vi "mislanius_time_add.vi"(8 "error in (no error)":errorcluster, 10 "Cluster out":T1={"connection reference"=refnum, "Net Avai time (Min)"=0, "pLAN dATE datA"=[], "Data by plan date, shift, product"=[], "BreakDownd Data"=[], "Raw rejection Data"=[], "mislanius times shift 1"={"Lunch Time From"=timestamp(0 s since 1904-01-01), "Lunch Time To"=timestamp(0 s since 1904-01-01), "Tea Time From"=timestamp(0 s since 1904-01-01), "Tea Time To"=timestamp(0 s since 1904-01-01), "Clean Time From"=timestamp(0 s since 1904-01-01), "Clean Time To"=timestamp(0 s since 1904-01-01), "Meeting Time From"=timestamp(0 s since 1904-01-01), "Meeting Time To"=timestamp(0 s since 1904-01-01), "Dev/Other Time From"=timestamp(0 s since 1904-01-01), "Dev/Other Time To"=timestamp(0 s since 1904-01-01), "Meeting"=FALSE, "Dev/Other"=TRUE}, "mislanius times shift 2"={"Lunch Time From"=timestamp(0 s since 1904-01-01), "Lunch Time To"=timestamp(0 s since 1904-01-01), "Tea Time From"=timestamp(0 s since 1904-01-01), "Tea Time To"=timestamp(0 s since 1904-01-01), "Clean Time From"=timestamp(0 s since 1904-01-01), "Clean Time To"=timestamp(0 s since 1904-01-01), "Meeting Time From"=timestamp(0 s since 1904-01-01), "Meeting Time To"=timestamp(0 s since 1904-01-01), "Dev/Other Time From"=timestamp(0 s since 1904-01-01), "Dev/Other Time To"=timestamp(0 s since 1904-01-01), "Meeting"=FALSE, "Dev/Other"=TRUE}} {"mislanius times shift 2"."Lunch Time From" format="%<%.X %x>T"; "mislanius times shift 2"."Lunch Time To" format="%<%.X %x>T"; "mislanius times shift 2"."Tea Time From" format="%<%.X %x>T"; "mislanius times shift 2"."Tea Time To" format="%<%.X %x>T"; "mislanius times shift 2"."Clean Time From" format="%<%.X %x>T"; "mislanius times shift 2"."Clean Time To" format="%<%.X %x>T"; "mislanius times shift 2"."Meeting Time From" format="%<%.X %x>T"; "mislanius times shift 2"."Meeting Time To" format="%<%.X %x>T"; "mislanius times shift 2"."Dev/Other Time From" format="%<%.X %x>T"; "mislanius times shift 2"."Dev/Other Time To" format="%<%.X %x>T"; "mislanius times shift 1"."Lunch Time From" format="%<%.X %x>T"; "mislanius times shift 1"."Lunch Time To" format="%<%.X %x>T"; "mislanius times shift 1"."Tea Time From" format="%<%.X %x>T"; "mislanius times shift 1"."Tea Time To" format="%<%.X %x>T"; "mislanius times shift 1"."Clean Time From" format="%<%.X %x>T"; "mislanius times shift 1"."Clean Time To" format="%<%.X %x>T"; "mislanius times shift 1"."Meeting Time From" format="%<%.X %x>T"; "mislanius times shift 1"."Meeting Time To" format="%<%.X %x>T"; "mislanius times shift 1"."Dev/Other Time From" format="%<%.X %x>T"; "mislanius times shift 1"."Dev/Other Time To" format="%<%.X %x>T"}, 11 "Shift":string(combo)="2") -> (0 "error out":errorcluster, 2 "Split DT time":u32[](array[numeric]), 3 "Total mis time":i32)   [LabVIEW 2017]
uses:
  Controls/OE_screen_cluster.ctl
  <vilib>/addons/database/Connection.llb/Conn ObjectReference.ctl
  <vilib>/addons/database/NI_Database_API.lvlib
panel:
  out "Lunch time 2":i32
  out "tea time 2":i32
  out "clean time 2":i32
  out "meeting time 2":i32
  out "Dev/other time 2":i32
  out "Dev/other time":i32
  out "meeting time":i32
  out "clean time":i32
  out "tea time":i32
  out "Lunch time":i32
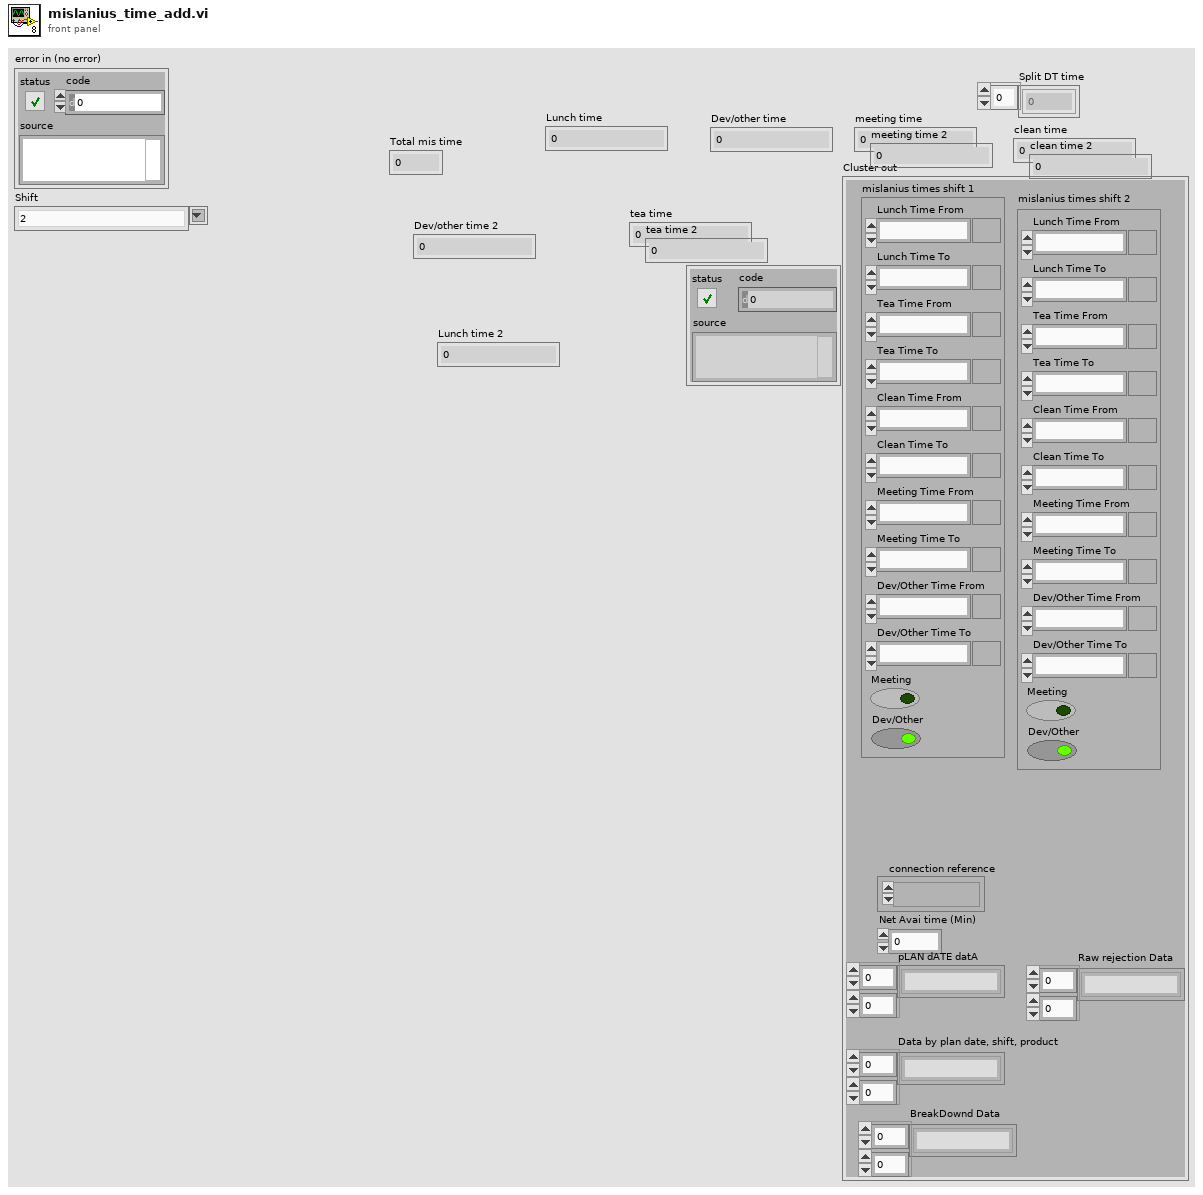
[diagram p1: front panel]
types:
  T1 = typedef "OE_screen_cluster.ctl" = cluster{"connection reference":T2, "Net Avai time (Min)":i32, "pLAN dATE datA":string[][], "Data by plan date, shift, product":string[][], "BreakDownd Data":string[][], "Raw rejection Data":string[][], "mislanius times shift 1":cluster{"Lunch Time From":timestamp, "Lunch Time To":timestamp, "Tea Time From":timestamp, "Tea Time To":timestamp, "Clean Time From":timestamp, "Clean Time To":timestamp, "Meeting Time From":timestamp, "Meeting Time To":timestamp, "Dev/Other Time From":timestamp, "Dev/Other Time To":timestamp, "Meeting":bool, "Dev/Other":bool}, "mislanius times shift 2":cluster{"Lunch Time From":timestamp, "Lunch Time To":timestamp, "Tea Time From":timestamp, "Tea Time To":timestamp, "Clean Time From":timestamp, "Clean Time To":timestamp, "Meeting Time From":timestamp, "Meeting Time To":timestamp, "Dev/Other Time From":timestamp, "Dev/Other Time To":timestamp, "Meeting":bool, "Dev/Other":bool}}
  T2 = typedef "NI_Database_API.lvlib/Conn ObjectReference.ctl" = refnum<k1>
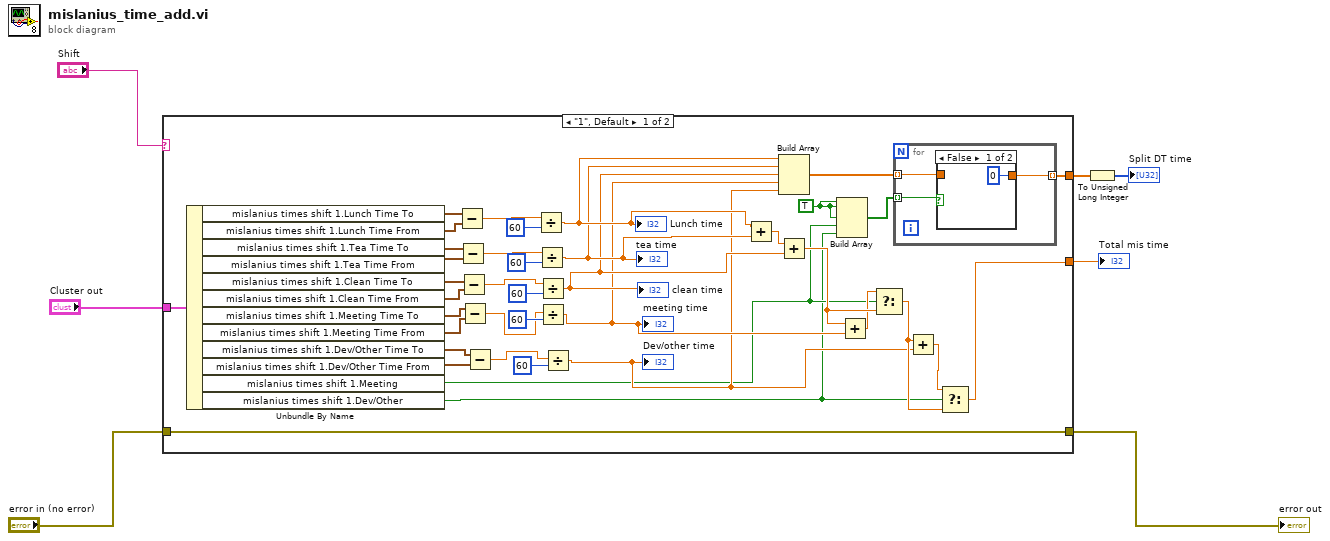
[diagram p0: block diagram]
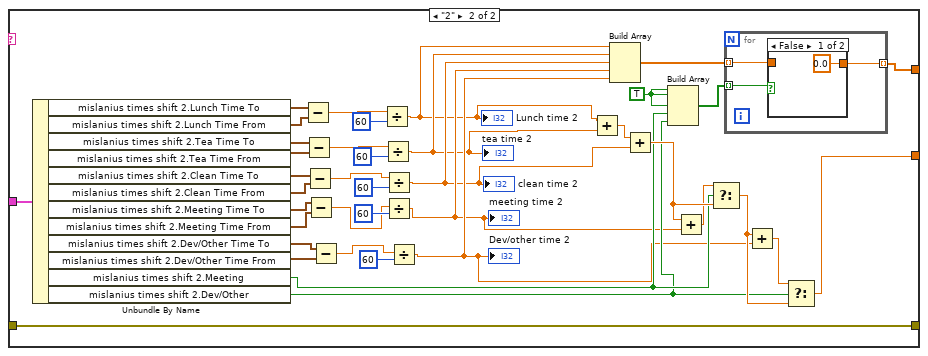
[diagram p3: hidden frame]
diagram:
  n1 = case shown="\"1\", Default" "Shift" {
    tunnel: [w20 w64] -> w7
    tunnel: "Cluster out" -> [w24 w68]
    tunnel: [w19 w63] -> w4
    tunnel: "error in (no error)" -> [w19 w63]
    tunnel: [w8 w60] -> w2
    frame "1", Default {
      w12 = TRUE
      n2 = Unbundle By Name(w24) -> ("mislanius times shift 1.Lunch Time To"=w44:timestamp, "mislanius times shift 1.Lunch Time From"=w43:timestamp, "mislanius times shift 1.Tea Time To"=w42:timestamp, "mislanius times shift 1.Tea Time From"=w41:timestamp, "mislanius times shift 1.Clean Time To"=w37:timestamp, "mislanius times shift 1.Clean Time From"=w36:timestamp, "mislanius times shift 1.Meeting Time To"=w33:timestamp, "mislanius times shift 1.Meeting Time From"=w32:timestamp, "mislanius times shift 1.Dev/Other Time To"=w28:timestamp, "mislanius times shift 1.Dev/Other Time From"=w27:timestamp, "mislanius times shift 1.Meeting"=w11:bool, "mislanius times shift 1.Dev/Other"=w10:bool)
      n3 = Subtract(x=w44, y=w43) -> (x-y=w46:dbl)
      n4 = Subtract(x=w42, y=w41) -> (x-y=w39:dbl)
      n5 = Subtract(x=w37, y=w36) -> (x-y=w34:dbl)
      n6 = Subtract(x=w33, y=w32) -> (x-y=w31:dbl)
      n7 = Subtract(x=w28, y=w27) -> (x-y=w30:dbl)
      n8 = Divide(x=w46, y=60) -> (x/y=w18:dbl)
      "Lunch time" <- w18
      n9 = Divide(x=w39, y=60) -> (x/y=w17:dbl)
      "tea time" <- w17
      n10 = Divide(x=w34, y=60) -> (x/y=w16:dbl)
      "clean time" <- w16
      n11 = Divide(x=w31, y=60) -> (x/y=w15:dbl)
      "meeting time" <- w15
      n12 = Divide(x=w30, y=60) -> (x/y=w14:dbl)
      "Dev/other time" <- w14
      n13 = Add(x=w18, y=w17) -> (x+y=w26:dbl)
      n14 = Build Array(w18, w17, w16, w15, w14) -> (w13:dbl[])
      n15 = Add(x=w26, y=w16) -> (x+y=w25:dbl)
      n16 = Build Array(w12, w12, w12, w11, w10) -> (w9:bool[])
      n17 = Add(x=w25, y=w15) -> (x+y=w23:dbl)
      n18 = Select(t=w23, s=w11, f=w25) -> (s? t:f=w21:dbl)
      n19 = for {
        tunnel: w13 -> [w47] mode=indexing
        tunnel: w9 -> [w49] mode=indexing
        tunnel: [w48] -> w8 mode=indexing
        n20 = case shown="False" w49 {
          tunnel: [0 w51] -> w48
          tunnel: w47 -> [_ w51]
          frame False {
          }
          frame True {
          }
        }
      }
      n21 = Add(x=w21, y=w14) -> (x+y=w22:dbl)
      n22 = Select(t=w22, s=w10, f=w21) -> (s? t:f=w20:dbl)
    }
    frame "2" {
      w61 = TRUE
      n23 = Unbundle By Name(w68) -> ("mislanius times shift 2.Lunch Time To"=w88:timestamp, "mislanius times shift 2.Lunch Time From"=w87:timestamp, "mislanius times shift 2.Tea Time To"=w86:timestamp, "mislanius times shift 2.Tea Time From"=w85:timestamp, "mislanius times shift 2.Clean Time To"=w81:timestamp, "mislanius times shift 2.Clean Time From"=w80:timestamp, "mislanius times shift 2.Meeting Time To"=w77:timestamp, "mislanius times shift 2.Meeting Time From"=w76:timestamp, "mislanius times shift 2.Dev/Other Time To"=w72:timestamp, "mislanius times shift 2.Dev/Other Time From"=w71:timestamp, "mislanius times shift 2.Meeting"=w59:bool, "mislanius times shift 2.Dev/Other"=w58:bool)
      n24 = Subtract(x=w88, y=w87) -> (x-y=w90:dbl)
      n25 = Subtract(x=w86, y=w85) -> (x-y=w83:dbl)
      n26 = Subtract(x=w81, y=w80) -> (x-y=w78:dbl)
      n27 = Subtract(x=w77, y=w76) -> (x-y=w75:dbl)
      n28 = Subtract(x=w72, y=w71) -> (x-y=w74:dbl)
      n29 = Divide(x=w90, y=60) -> (x/y=w53:dbl)
      "Lunch time 2" <- w53
      n30 = Divide(x=w83, y=60) -> (x/y=w54:dbl)
      "tea time 2" <- w54
      n31 = Divide(x=w78, y=60) -> (x/y=w55:dbl)
      "clean time 2" <- w55
      n32 = Divide(x=w75, y=60) -> (x/y=w56:dbl)
      "meeting time 2" <- w56
      n33 = Divide(x=w74, y=60) -> (x/y=w57:dbl)
      "Dev/other time 2" <- w57
      n34 = Add(x=w53, y=w54) -> (x+y=w70:dbl)
      n35 = Build Array(w53, w54, w55, w56, w57) -> (w52:dbl[])
      n36 = Add(x=w70, y=w55) -> (x+y=w69:dbl)
      n37 = Build Array(w61, w61, w61, w59, w58) -> (w62:bool[])
      n38 = Add(x=w69, y=w56) -> (x+y=w67:dbl)
      n39 = Select(t=w67, s=w59, f=w69) -> (s? t:f=w65:dbl)
      n40 = for {
        tunnel: w52 -> [w91] mode=indexing
        tunnel: w62 -> [w93] mode=indexing
        tunnel: [w92] -> w60 mode=indexing
        n41 = case shown="False" w93 {
          tunnel: [0.0 w95] -> w92
          tunnel: w91 -> [_ w95]
          frame False {
          }
          frame True {
          }
        }
      }
      n42 = Add(x=w65, y=w57) -> (x+y=w66:dbl)
      n43 = Select(t=w66, s=w58, f=w65) -> (s? t:f=w64:dbl)
    }
  }
  "Total mis time" <- w7
  "error out" <- w4
  n44 = To Unsigned Long Integer(number=w2) -> (unsigned 32bit integer=→"Split DT time":u32[])
